vi "CSTK_MCListbox_Designer_MoveUpColHdr.vi"(7 "表头属性列表输入":refnum<vi>, 8 "错误输入（无错误）":errorcluster, 9 "Selected Index":i32, 10 "MCListbox引用句柄":refnum<vi>, 11 "VI输入":refnum<vi>) -> (0 "错误输出":errorcluster, 3 "VI输出":refnum<vi>)   [LabVIEW 2015, in "CSTK_MCListbox Designer.lvlib"]
uses:
  CSTK_MCListbox Designer.lvlib
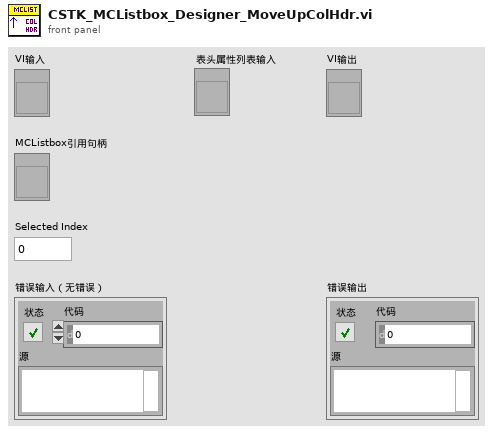
[diagram p1: front panel]
types:
  T1 = typedef "CSTK_MCListbox Designer.lvlib/_CSTK_MCListbox_Designer_ColHdr_Selected.ctl" = cluster{"选择":bool, "表头属性":T2}
  T2 = typedef "CSTK_MCListbox Designer.lvlib/_CSTK_MCListbox_Designer_ColHdr.ctl" = cluster{"列名称":string, "单元格宽度":u32, "粗体":bool, "斜体":bool, "对齐":enum16{"Left", "Center", "Right"}}
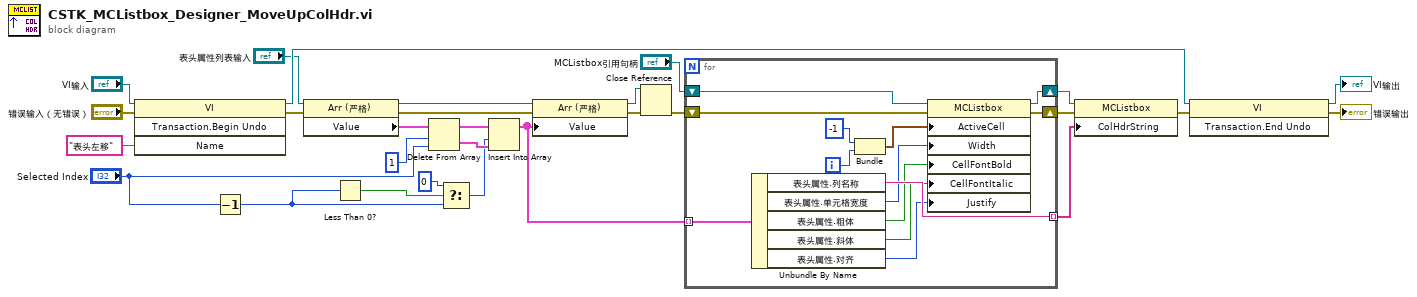
[diagram p0: block diagram]
diagram:
  n1 = invoke class="VI" method="Transaction.Begin Undo"(reference="VI输入", error in="错误输入（无错误）", "Name"="表头左移" ("名称")) -> (reference out=w15:refnum<vi>, error out=w23:errorcluster)  [unwired: 1 in, 2 out]
  n2 = Decrement(x="Selected Index") -> (x-1=w10:i32)
  n3 = property on="属性节点" class="Arr (严格)"(reference="表头属性列表输入", error in=w23) -> (reference out=w6:refnum<vi>, error out=w4:errorcluster, "Value"=w24:T1[])
  n4 = Less Than 0?(x=w10) -> (x < 0?=w12:bool)
  n5 = Delete From Array(array=w24, length=1 ("长度"), index="Selected Index") -> (deleted portion=w8:T1[], array with subset deleted=w13:T1[])
  n6 = Select(t=0 ("x-1"), s=w12, f=w10) -> (s? t:f=w7:i32)
  n7 = Insert Into Array(array=w13, index=w7, new element=w8) -> (w3:T1[])
  n8 = property on="属性节点" class="Arr (严格)"(reference=w6, error in=w4, "Value"=w3) -> (reference out=w5:refnum<vi>, error out=w2:errorcluster)
  n9 = Close Reference(reference=w5, error in (no error)=w2) -> (error out=w14:errorcluster)
  n10 = for {
    tunnel: w3 -> [w39] mode=indexing
    tunnel: [w38] -> w27 mode=indexing
    shift-right: [w35] -> w25
    shift-left: "MCListbox引用句柄" -> [w36]
    shift-right: [w30] -> w26
    shift-left: w14 -> [w31]
    i -> [w40]
    n11 = Unbundle By Name(w39) -> ("表头属性.列名称"=w38:string, "表头属性.单元格宽度"=w34:u32, "表头属性.粗体"=w33:bool, "表头属性.斜体"=w29:bool, "表头属性.对齐"=w32:enum16{"Left", "Center", "Right"})
    n12 = Bundle(-1, w40) -> (w37:cluster{i32, i32})  [unwired: 1 in]
    n13 = property class="MCListbox"(reference=w36, error in=w31, "ActiveCell"=w37, "Width"=w34, "CellFontBold"=w33, "CellFontItalic"=w29, "Justify"=w32) -> (reference out=w35:refnum<vi>, error out=w30:errorcluster)
  }
  n14 = property class="MCListbox"(reference=w25, error in=w26, "ColHdrString"=w27) -> (error out=w28:errorcluster)  [unwired: 1 out]
  n15 = invoke class="VI" method="Transaction.End Undo"(reference=w15, error in=w28) -> (reference out=→"VI输出":refnum<vi>, error out=→"错误输出":errorcluster)  [unwired: 1 in, 1 out]
